vi "Smoother.vi"(8 "tolerance":dbl, 9 "B":dbl, 10 "A":dbl, 11 "Path":cluster{"x":dbl, "y":dbl}[](array[cluster])=[{"x"=0.0, "y"=0.0}, {"x"=0.0, "y"=46.0}, {"x"=77.25, "y"=97.5}]) -> (3 "Smooth Path":cluster{"x":dbl, "y":dbl}[](array[cluster])=[{"x"=0.0, "y"=0.0}, {"x"=0.0, "y"=46.0}, {"x"=77.25, "y"=97.5}])   [LabVIEW 2016]
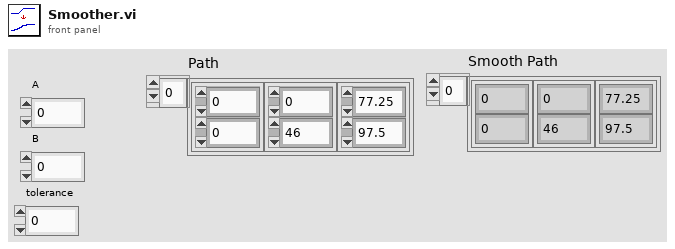
[diagram p1: front panel]
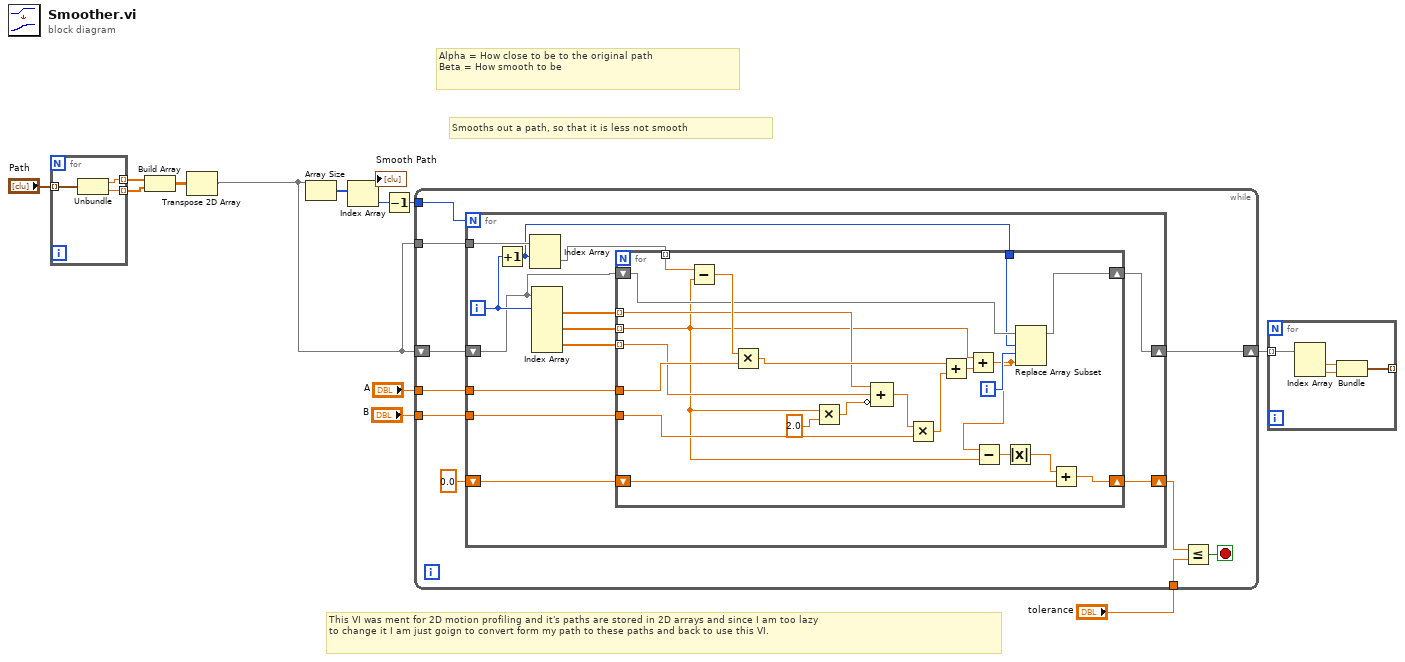
[diagram p0: block diagram]
diagram:
  # "Smooths out a path, so that it is less not smooth"
  # "Alpha = How close to be to the original path\nBeta = How smooth to be"
  # "This VI was ment for 2D motion profiling and it's paths are stored in 2D arrays and since I am too lazy\nto change it I am just goign to convert form my path to these paths and back to use this VI."
  n1 = for {
    tunnel: "Path" -> [w15] mode=indexing
    tunnel: [w14] -> w6 mode=indexing
    tunnel: [w13] -> w5 mode=indexing
    n2 = Unbundle(w15) -> ("x"=w14:dbl, "y"=w13:dbl)
  }
  n3 = Build Array(w6, w5) -> (w4:dbl[][])
  n4 = Transpose 2D Array(2D array=w4) -> (transposed array=w2:dbl[][])
  n5 = Array Size(array=w2) -> (size(s)=w12:i32[])
  n6 = Index Array(array=w12) -> (element=w11:i32)  [unwired: 1 in]
  n7 = Decrement(x=w11) -> (x-1=w10:i32)
  n8 = while {
    tunnel: w10 -> [w25]
    tunnel: "A" -> [w24]
    tunnel: "B" -> [w23]
    tunnel: w2 -> [w22]
    shift-right: [w20] -> w1
    shift-left: w2 -> [w21]
    tunnel: "tolerance" -> [w19]
    stop <- w18 stop-if-true
    n9 = for {
      N: w25 -> [_]
      tunnel: w24 -> [w38]
      tunnel: w23 -> [w37]
      tunnel: w22 -> [w35]
      shift-right: [w28] -> w20
      shift-left: w21 -> [w30]
      shift-right: [w27] -> w16
      shift-left: 0.0 -> [w26]
      i -> [w34]
      n10 = Increment(x=w34) -> (x+1=w29:i32)
      n11 = Index Array(array=w35, index (row)=w29) -> (element=w33:dbl[])  [unwired: 1 in]
      n12 = Index Array(array=w30, index (row) #1=w34) -> (element #1=w32:dbl[], element #2=w36:dbl[], element #3=w31:dbl[])  [unwired: 5 in]
      n13 = for {
        tunnel: w36 -> [w43] mode=indexing
        tunnel: w38 -> [w60]
        tunnel: w37 -> [w56]
        tunnel: w33 -> [w59] mode=indexing
        tunnel: w32 -> [w55] mode=indexing
        tunnel: w31 -> [w54] mode=indexing
        tunnel: w29 -> [w46]
        shift-right: [w45] -> w28
        shift-left: w30 -> [w48]
        shift-right: [w41] -> w27
        shift-left: w26 -> [w40]
        i -> [w47]
        n14 = Subtract(x=w59, y=w43) -> (x-y=w58:dbl)
        n15 = Multiply(x=w58, y=w60) -> (x*y=w57:dbl)
        n16 = Multiply(x=w43, y=2.0) -> (x*y=w53:dbl)
        n17 = Compound Arithmetic op=ADD(w55, w54, invert w53) -> (w51:dbl)
        n18 = Multiply(x=w51, y=w56) -> (x*y=w50:dbl)
        n19 = Add(x=w57, y=w50) -> (x+y=w49:dbl)
        n20 = Add(x=w43, y=w49) -> (x+y=w44:dbl)
        n21 = Subtract(x=w44, y=w43) -> (x-y=w42:dbl)
        n22 = Absolute Value(x=w42) -> (abs(x)=w39:dbl)
        n23 = Replace Array Subset(array=w48, new element=w44, index (row)=w46, index (col)=w47) -> (w45:dbl[][])
        n24 = Add(x=w39, y=w40) -> (x+y=w41:dbl)
      }
    }
    n25 = Less Or Equal?(x=w16, y=w19) -> (x <= y?=w18:bool)
  }
  n26 = for {
    tunnel: w1 -> [w64] mode=indexing
    tunnel: [w61] -> _ mode=indexing
    n27 = Index Array(array=w64) -> (element #1=w63:dbl, element #2=w62:dbl)  [unwired: 2 in]
    n28 = Bundle("y"=w63, "y"=w62) -> (w61:cluster{"y":dbl, "y":dbl})  [unwired: 1 in]
  }
